vi "e.gate ASCII Query.vi"(8 "error in (no error)":errorcluster, 10 "Command":string, 11 "connection ID In":refnum<k5>) -> (0 "error out":errorcluster, 2 "Response":string, 3 "connection ID Out":refnum<k5>)   [LabVIEW 2016]
doc: "<B>AMC - Analytik & Messtechnik GmbH Chemnitz</B>\n\nLabVIEW Drivers for e.gate / e.pac series from Gantner Instruments\n\nThis VI is a driver subroutine and should not be used in an application. It assembles a module command string out of the parameters and writes it to the TCP/IP interface specified in <B>connection ID In</B>. Followed by the module command the response is read from the interface and provided in <B>Response</B>."
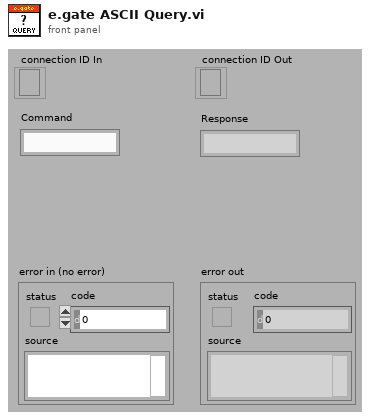
[diagram p1: front panel]
types:
  T1 = enum16{"Standard", "Buffered", "CRLF", "Immediate"}
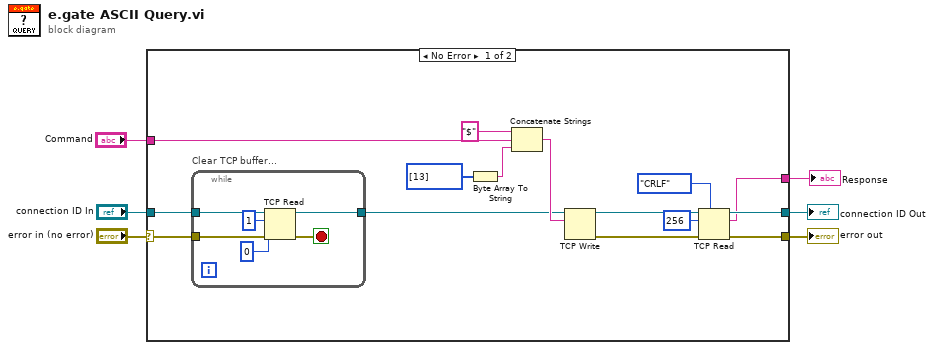
[diagram p0: block diagram]
diagram:
  n1 = case shown="No Error" "error in (no error)" {
    selector: "error in (no error)" -> [w9 w28]
    tunnel: "connection ID In" -> [w8 w29]
    tunnel: [w14 w29] -> w4
    tunnel: [w13 w28] -> w3
    tunnel: "Command" -> [w20 _]
    tunnel: [w12 _] -> w1
    frame No Error {
      n2 = while "Clear TCP buffer..." {
        tunnel: w9 -> [w26]
        tunnel: w8 -> [w27]
        tunnel: [w24] -> w7
        stop <- w25 stop-if-true
        n3 = TCP Read(connection ID=w27, bytes to read=1, error in (no error)=w26, 9:0 ("timeout ms (25000)")) -> (connection ID out=w24:refnum<k5>, error out=w25:errorcluster)  [unwired: 2 out]
      }
      n4 = Byte Array To String(unsigned byte array=u8[] [13]) -> (string=w18:string)
      n5 = Concatenate Strings("$" ("string"), w20, w18) -> (w17:string)
      n6 = TCP Write(connection ID=w7, data in=w17) -> (connection ID out=w15:refnum<k5>, error out=w16:errorcluster)  [unwired: 1 in, 2 out]
      n7 = TCP Read(connection ID=w15, bytes to read=256, error in (no error)=w16, 7:T1."CRLF" ("mode (standard)")) -> (connection ID out=w14:refnum<k5>, data out=w12:string, error out=w13:errorcluster)  [unwired: 1 out]
    }
    frame Error {
    }
  }
  "error out" <- w3
  "connection ID Out" <- w4
  "Response" <- w1
